vi "DiffDriveTrainSim_CreateKitbotSim_EstMassMOI.vi"(6 "MeasurementStdDev":T4, 8 "TrackWidth_M":dbl, 9 "Wheelsize":T1, 10 "ToughBoxMiniGear":T2, 11 "ToughBoxMiniMotor":T3) -> (0 "Size Coerced":bool, 3 "DiffDriveTrainSim":T5 {"m_Motor"."Kt_NMPerAmp" format="%13.5p"; "m_Motor"."Kv_RadPerSecPerVolt" format="%13.5p"; "m_Motor"."R_Ohms" format="%13.5p"; "m_Motor"."FreeSpeed_RadPerSec" format="%13.5p"; "m_Motor"."FreeCurrent_Amps" format="%13.5p"; "m_Motor"."StallCurrent_Amps" format="%13.5p"; "m_Motor"."StallTorque_NM" format="%13.5p"; "m_Motor"."nominalVoltage_Volts" format="%13.5p"})   [LabVIEW 2019, in "Trajectory_Library.lvlib"]
doc: "Creates a new LINEAR SYSTEM data cluster with the specified values. \n\n\nInputs: \n - XXX -- XXX.\n\nOutputs:\n - XXX -- XXX."
uses:
  Trajectory_Library.lvlib
  DIFF_DRIVE_TRAIN_SIM.ctl
  LINEAR_SYSTEM.ctl
  <vilib>/Analysis/Matrix/Datatypes/RealMatrix.ctl
  DCMOTOR.CTL
  DIFF_DRIVE_ToughBoxMini_MotorChoice_ENUM.ctl
  DIFF_DRIVE_ToughBoxMini_GearChoice_ENUM.ctl
  DIFF_DRIVE_KitBot_WheelSize_ENUM.ctl
  Conv_Inches_Meters.vi
  <vilib>/Analysis/Matrix/NI_Matrix.lvlib
panel:
  # "<1, 1>"
  # "<States, 1>"
  # "<Outputs, 1>"
  # "<Inputs, 1>"
  # "<Outputs, 1>"
  # "<States,States>"
  # "<States,Inputs>"
  # "<Outputs,States>"
  # "<Outputs,Inputs>"
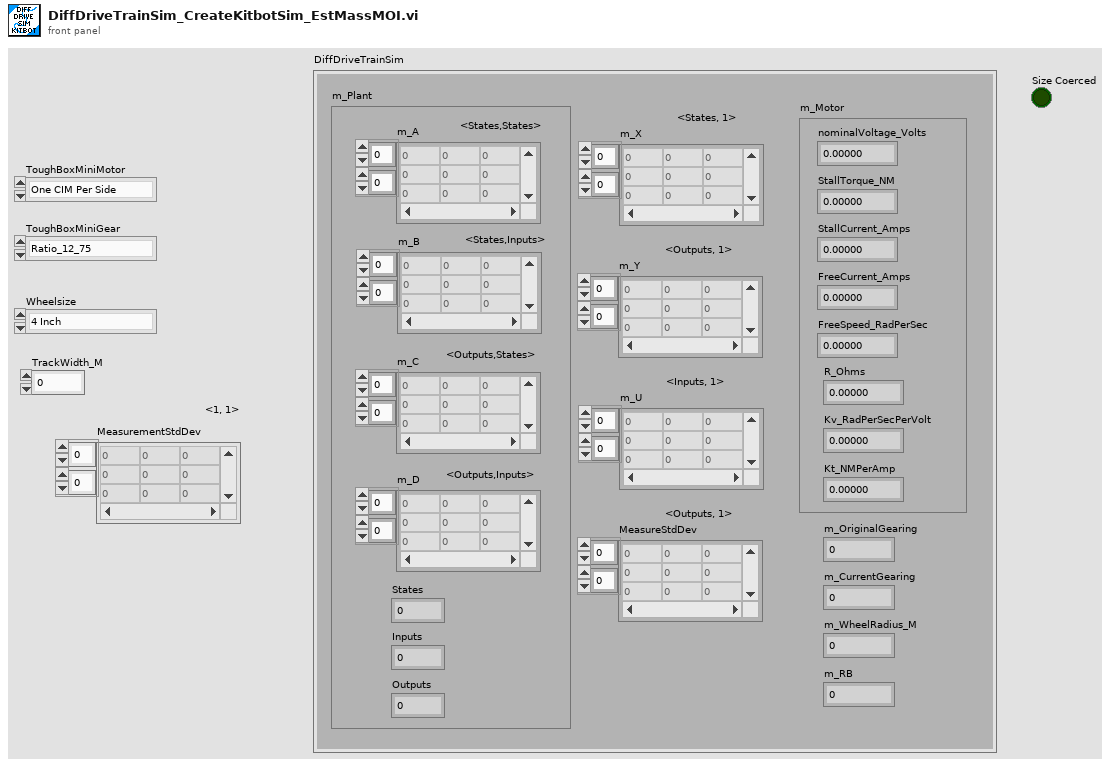
[diagram p1: front panel]
types:
  T1 = typedef "Trajectory_Library.lvlib/DIFF_DRIVE_KitBot_WheelSize_ENUM.ctl" = enum16{"4 Inch", "6 Inch", "8 Inch", "10 Inch"}
  T2 = typedef "Trajectory_Library.lvlib/DIFF_DRIVE_ToughBoxMini_GearChoice_ENUM.ctl" = enum16{"Ratio_12_75", "Ratio_10_71", "Ratio_8_45", "Ratio_7_31", "Ratio_5_95"}
  T3 = typedef "Trajectory_Library.lvlib/DIFF_DRIVE_ToughBoxMini_MotorChoice_ENUM.ctl" = enum16{"One CIM Per Side", "Two CIM Per Side", "One MiniCIM Per Side", "Two Mini CIM Per Side", "Two Falcon Per Side", "Two NEO Per Side"}
  T4 = typedef "NI_Matrix.lvlib/RealMatrix.ctl" = dbl[][]
  T5 = typedef "Trajectory_Library.lvlib/DIFF_DRIVE_TRAIN_SIM.ctl" = cluster{"m_Plant":T6, "m_X":T4, "m_Y":T4, "m_U":T4, "MeasureStdDev":T4, "m_Motor":T7, "m_OriginalGearing":dbl, "m_CurrentGearing":dbl, "m_WheelRadius_M":dbl, "m_RB":dbl}
  T6 = typedef "Trajectory_Library.lvlib/LINEAR_SYSTEM.ctl" = cluster{"m_A":T4, "m_B":T4, "m_C":T4, "m_D":T4, "States":i32, "Inputs":i32, "Outputs":i32}
  T7 = typedef "Trajectory_Library.lvlib/DCMOTOR.CTL" = cluster{"nominalVoltage_Volts":dbl, "StallTorque_NM":dbl, "StallCurrent_Amps":dbl, "FreeCurrent_Amps":dbl, "FreeSpeed_RadPerSec":dbl, "R_Ohms":dbl, "Kv_RadPerSecPerVolt":dbl, "Kt_NMPerAmp":dbl}
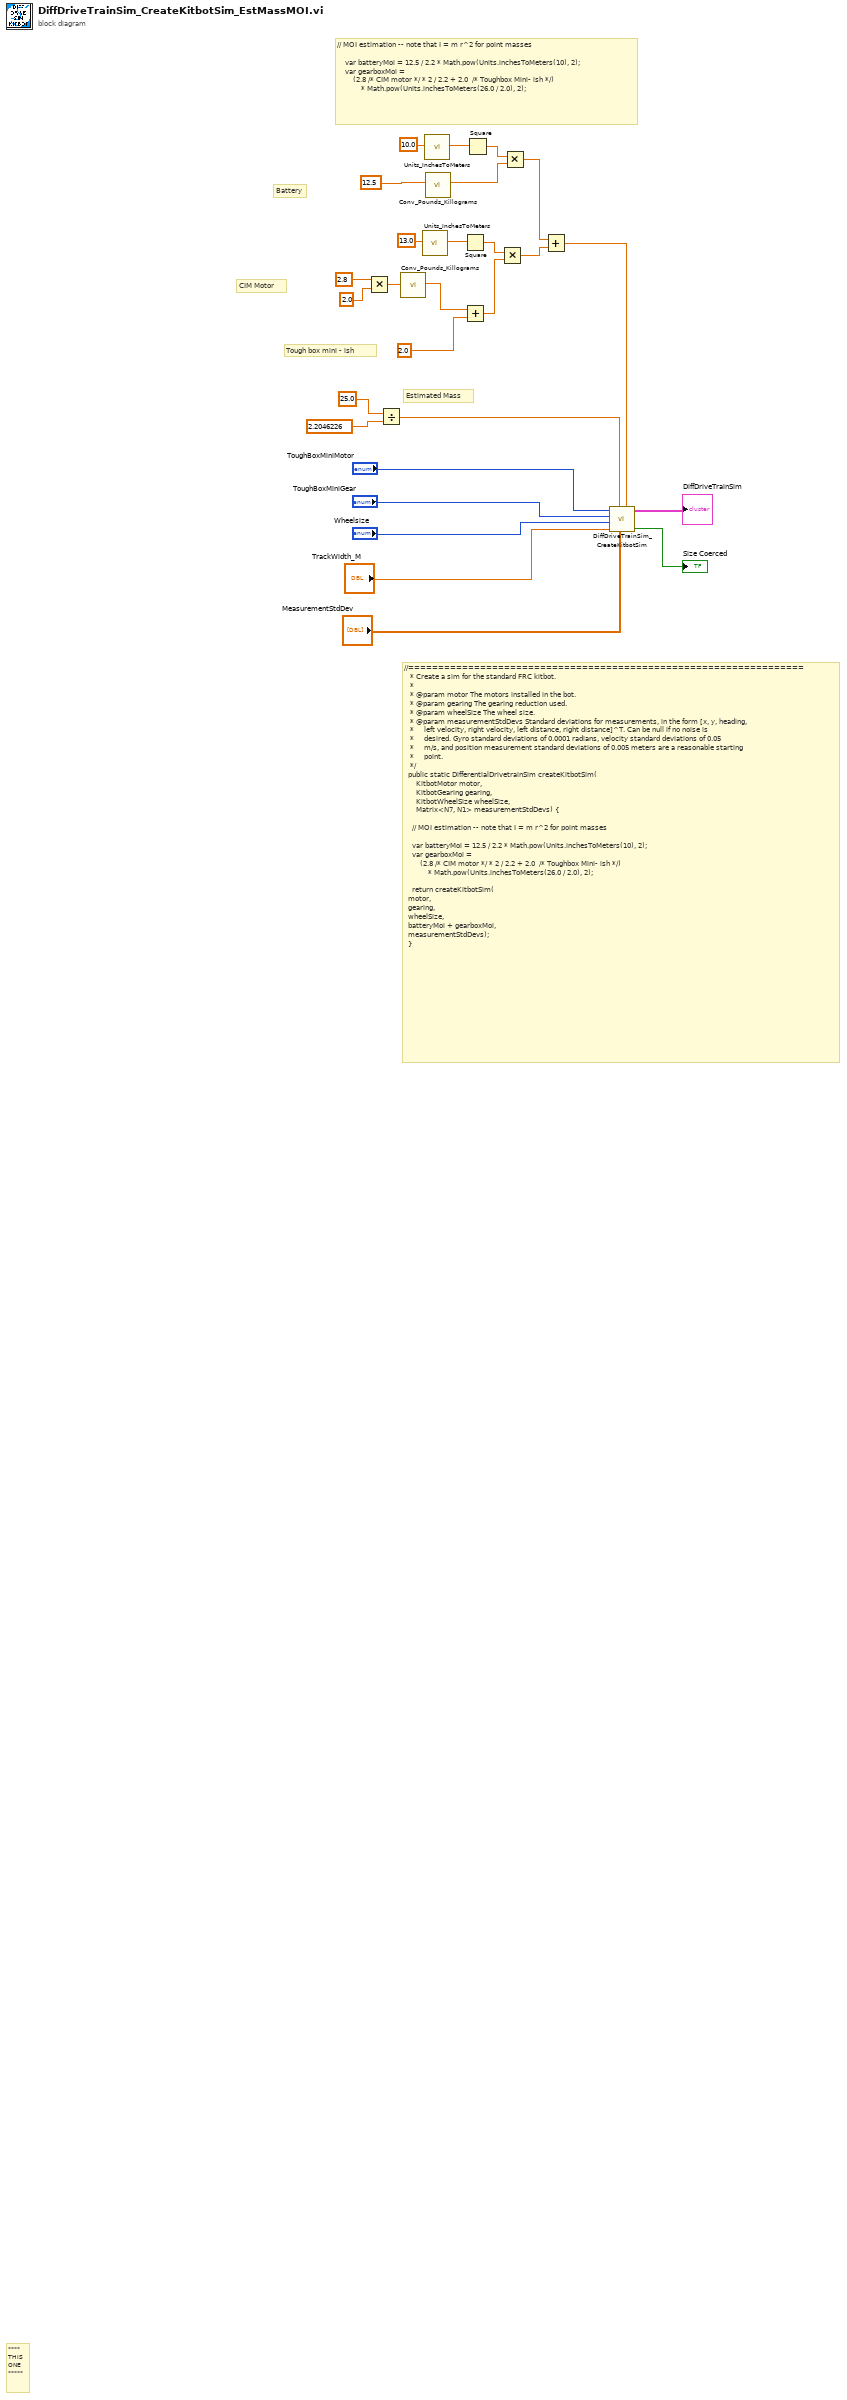
[diagram p0: block diagram]
diagram:
  # "Tough box mini - ish"
  # "Battery"
  # "CIM Motor"
  # "// MOI estimation -- note that I = m r^2 for point masses\n\n    var batteryMoi = 12.5 / 2.2 * Math.pow(Units.inchesToMeters(10), 2);\n    var gearboxMoi =\n        (2.8 /* CIM motor */ * 2 / 2.2 + 2.0 \t/* Toughbox Mini- ish */)\n            * Math.pow(Units.inchesToMeters(26.0 / 2.0), 2);"
  # "Estimated Mass"
  # "//==================================================================\n   * Create a sim for the standard FRC kitbot.\n   *\n   * @param motor The motors installed in the bot.\n   * @param gearing The gearing reduction used.\n   * @param wheelSize The wheel size.\n   * @param measurementStdDevs Standard deviations for measurements, in the form [x, y, heading,\n   *     left velocity, right velocity, left distance, right distance]^T. Can be null if no noise is\n   *     desired. Gyro standard deviations of 0.0001 radians, velocity standard deviations of 0.05\n   *     m/s, and position measurement standard deviations of 0.005 meters are a reasonable starting\n   *     point.\n   */\n  public static DifferentialDrivetrainSim createKitbotSim(\n      KitbotMotor motor,\n      KitbotGearing gearing,\n      KitbotWheelSize wheelSize,\n      Matrix<N7, N1> measurementStdDevs) {\n\n    // MOI estimation -- note that I = m r^2 for point masses\n\n    var batteryMoi = 12.5 / 2.2 * Math.pow(Units.inchesToMeters(10), 2);\n    var gearboxMoi =\n        (2.8 /* CIM motor */ * 2 / 2.2 + 2.0 \t/* Toughbox Mini- ish */)\n            * Math.pow(Units.inchesToMeters(26.0 / 2.0), 2);\n\n    return createKitbotSim(\n\t\tmotor, \n\t\tgearing, \n\t\twheelSize, \n\t\tbatteryMoi + gearboxMoi, \n\t\tmeasurementStdDevs);\n  }"
  # "****\nTHIS\nONE\n*****"
  n1 = Multiply(x=2.8, y=2.0) -> (x*y=w3:dbl)
  n2 = Divide(x=25.0, y=2.2046226) -> (x/y=w24:dbl)
  n3 = call "Conv_Pounds_Killograms.vi"("Pounds"=w3) -> ("Killograms"=w2:dbl)  [unwired: 10 in]
  n4 = call "Units_InchesToMeters.vi"("Inches"=13.0) -> ("Meters"=w11:dbl)  [unwired: 10 in]
  n5 = call "Units_InchesToMeters.vi"("Inches"=10.0) -> ("Meters"=w15:dbl)  [unwired: 10 in]
  n6 = call "Conv_Pounds_Killograms.vi"("Pounds"=12.5 ("x")) -> ("Killograms"=w5:dbl)  [unwired: 10 in]
  n7 = Square(x=w11) -> (x^2=w10:dbl)
  n8 = Add(x=w2, y=2.0) -> (x+y=w9:dbl)
  n9 = Square(x=w15) -> (x^2=w14:dbl)
  n10 = Multiply(x=w10, y=w9) -> (x*y=w8:dbl)
  n11 = Multiply(x=w14, y=w5) -> (x*y=w7:dbl)
  n12 = Add(x=w7, y=w8) -> (x+y=w6:dbl)
  n13 = call "DiffDriveTrainSim_CreateKitbotSim.vi"("j_KgM2"=w6, "MeasurementStdDev"="MeasurementStdDev", "Mass_Kg"=w24, "TrackWidth_M"="TrackWidth_M", "Wheelsize"="Wheelsize", "ToughBoxMiniGear"="ToughBoxMiniGear", "ToughBoxMiniMotor"="ToughBoxMiniMotor") -> ("Size Coerced"=→"Size Coerced":bool, "DiffDriveTrainSim"=→"DiffDriveTrainSim":T5)  [unwired: 3 in]
